vi "pf Close Port.vi"(8 "error in (no error)":errorcluster, 11 "iPort":i32) -> (0 "error out":errorcluster, 3 "function return":i32)   [LabVIEW 2012, in "Photonfocus_Toolkit.lvlib"]
doc: "PFCONFIG_API int pfClosePort(void);"
uses:
  <userlib>/Photonfocus Toolkit/Photonfocus_Toolkit.lvlib
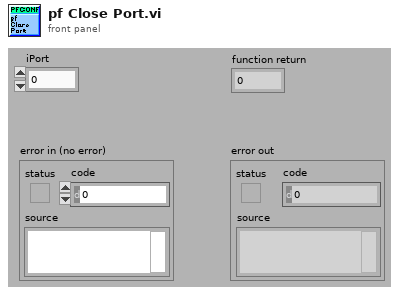
[diagram p1: front panel]
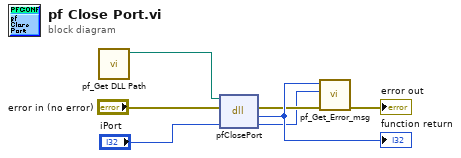
[diagram p0: block diagram]
diagram:
  n1 = call <userlib>:"pf_Get DLL Path.vi"() -> ("DLL path"=w3:path)  [unwired: 1 in, 10 out]
  n2 = dll-call lib="S:/Progetti/Photonfocus/Codice/DEV/PFConfig_lvlib/PFConfig.*" fn="pfClosePort"(path in=w3, error in="error in (no error)", "iPort"="iPort") -> (error out=w5:errorcluster, "return type"=w7:i32, "iPort"=w1:i32)  [unwired: 1 in, 1 out]
  "function return" <- w7
  n3 = call <userlib>:"pf_Get_Error_msg.vi"("error in (no error)"=w5, "iPort"=w1, "error code"=w7) -> ("error out"=→"error out":errorcluster)  [unwired: 8 out]
